vi "Simple Video Analyzer.vi"() -> ()   [LabVIEW 2013]
uses:
  _Type Defs/PhCon GS.ctl
  _Type Defs/PhCon Predefined Cines.ctl
  _Type Defs/PhFile InfName.ctl
  _Type Defs/PHCon IMRANGE.ctl
  _Type Defs/PhInt PhProcessImage Selectors.ctl
  <vilib>/Platform/browser.llb/Open URL in Default Browser (path).vi
  VRI.lvlib
  <vilib>/Analysis/NI_AALBase.lvlib
  _Type Defs/PhCon SDLO.ctl
panel:
  in  "Help":bool
  in  "Exp":dbl format="%#_g us"
  in  "Rate":dbl format="%#_g fps"
  in  "Res":string
  out "Model":string
  out "Image":picture
  out "Frame Brightness":string
  out "Frame":i32(slide) min=-186 max=10 step=1 scale=-2399.0..1999.0
  out "Progress":u8(slide) scale=0.0..100.0
  in  "Save":bool
  in  "Playback":bool
  in  "Trigger":bool
  in  "Record":bool
  out "Name":string
  out "Serial":u32
  in  "Camera Number":u32
  out "IP":string
  # "Simple Video Analyzer"
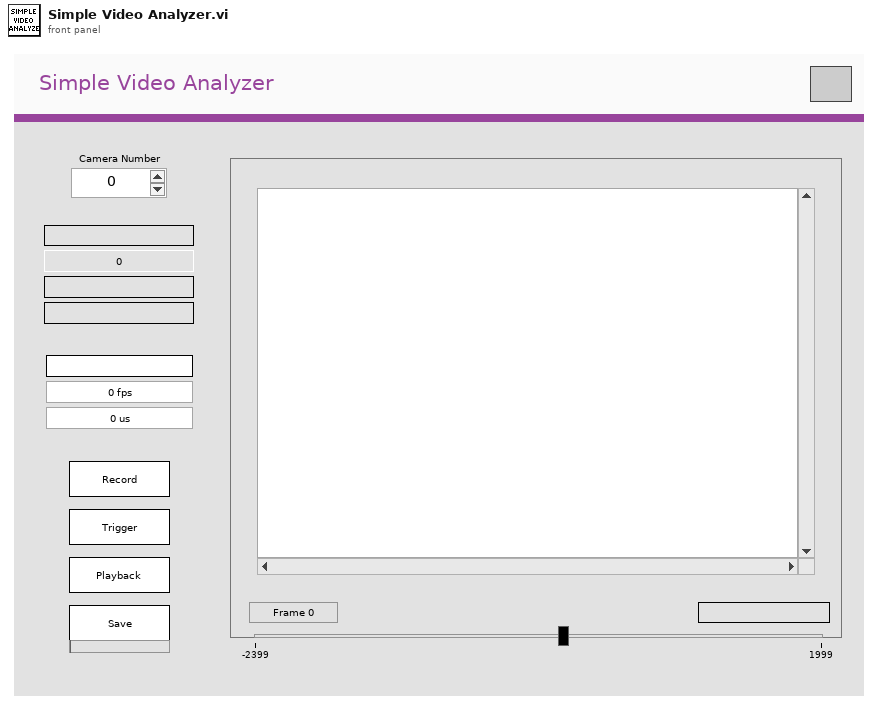
[diagram p1: front panel]
types:
  T1 = typedef "VRI.lvlib/PHCon IMRANGE.ctl" = cluster{"First":i32, "Cnt":u32}
  T2 = typedef "VRI.lvlib/PhCon SDLO.ctl" = u32
  T3 = typedef "VRI.lvlib/PhCon Predefined Cines.ctl" = i32
  T4 = typedef "VRI.lvlib/PhCon GS.ctl" = u16
  T5 = typedef "VRI.lvlib/PHCon ACQUIPARAMS.ctl" = cluster{"ImWidth":u32, "ImHeight":u32, "(deprecated)FrameRateInt":u32, "Exposure":u32, "EDRExposure":u32, "ImDelay":u32, "PTFrames":u32, "ImCount":u32, "SyncImaging":T6, "AutoExposure":u32, "AutoExpLevel":u32, "AutoExpSpeed":u32, "AutoExpRect":T7, "Recorded":bool, "TriggerTime":T8, "RecordedCount":u32, "FirstIm":i32, "FRPSteps":u32, "FRPImgNr":i32[], "FRPRate":u32[], "FRPExp":u32[], "Decimation":u32, "BitDepth":u32, "CamGainRed":u32, "CamGainGreen":u32, "CamGainBlue":u32, "CamGain":u32, "ShutterOff":bool, "CFA":T9, "CineName[256]":u8[], "Description[4096]":u8[], "FRPShape [16]":u32[], "dFrameRate":dbl}
  T6 = typedef "VRI.lvlib/PhCon SyncImaging.ctl" = enum32{"SYNC_INTERNAL", "SYNC_EXTERNAL", "SYNC_LOCKTOIRIG"}
  T7 = typedef "VRI.lvlib/Rect.ctl" = cluster{"X":i32, "Y":i32, "Width":i32, "Height":i32}
  T8 = typedef "VRI.lvlib/PHCon Time64.ctl" = cluster{"fractions":u32, "seconds":u32}
  T9 = typedef "VRI.lvlib/PhInt CFA.ctl" = cluster{"CFA":u32, "VRIV6 Mask":cluster{"TL_GRAY":bool, "TR_GRAY":bool, "BL_GRAY":bool, "BR_GRAY":bool}}
  T10 = typedef "VRI.lvlib/PhFile InfName.ctl" = u32
  T11 = typedef "VRI.lvlib/PhInt PhProcessImage Selectors.ctl" = u16
  T12 = typedef "VRI.lvlib/PhInt IH.ctl" = cluster{"biSize":u32, "biWidth":i32, "biHeight":i32, "biPlanes":u16, "biBitCount":u16, "biCompresssion":u32, "biSizeImage":u32, "biXPelsPerMeter":i32, "biYPelsPerMeter":i32, "biClrUsed":u32, "biClrImportant":u32, "BlackLevel":i32, "WhiteLevel":i32}
  T13 = typedef "VRI.lvlib/BITMAPINFOHEADER.ctl" = cluster{"biSize":u32, "biWidth":i32, "biHeight":i32, "biPlanes":u16, "biBitCount":u16, "biCompression":u32, "biSizeImage":u32, "biXPelsPerMeter":i32, "biYPelsPerMeter":i32, "biClrUsed":u32, "biClrImportant":u32}
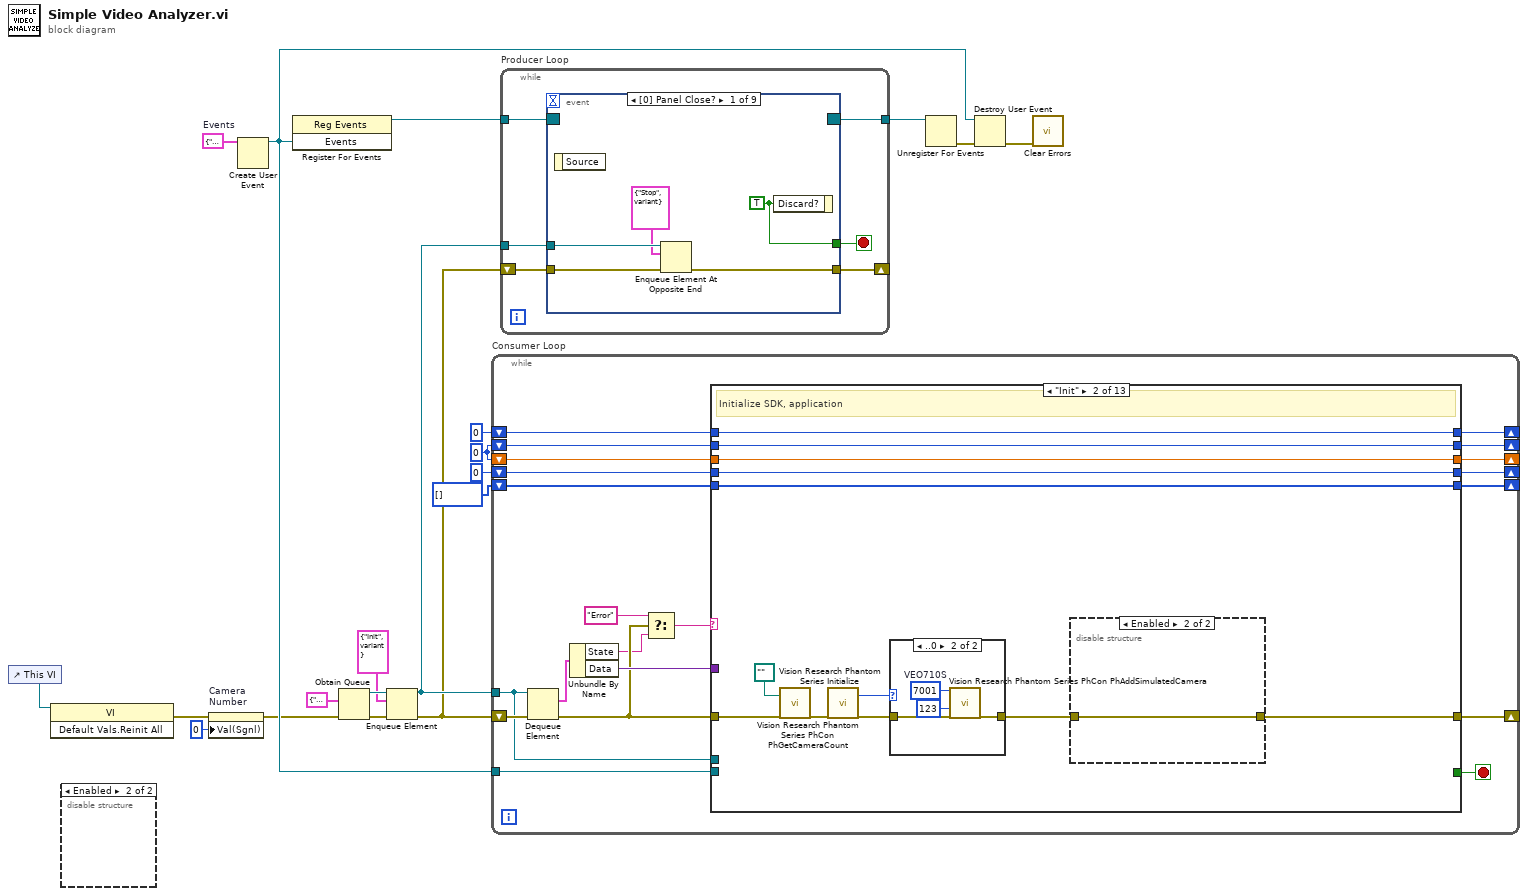
[diagram p0: block diagram]
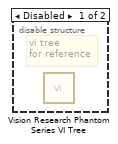
[diagram p2: hidden frame]
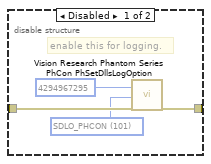
[diagram p5: hidden frame]
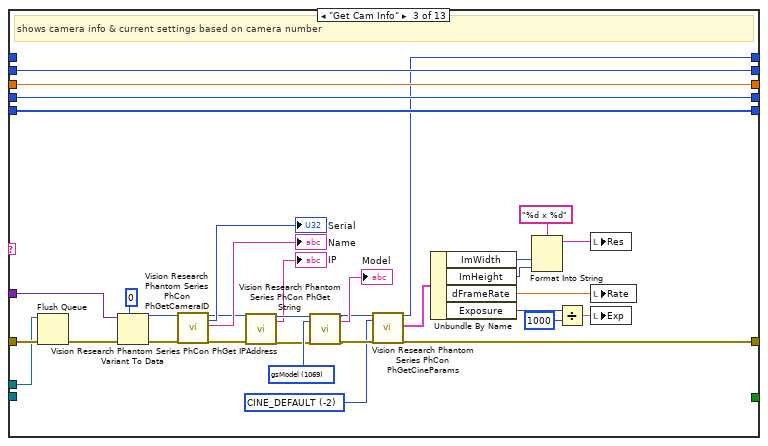
[diagram p6: hidden frame]
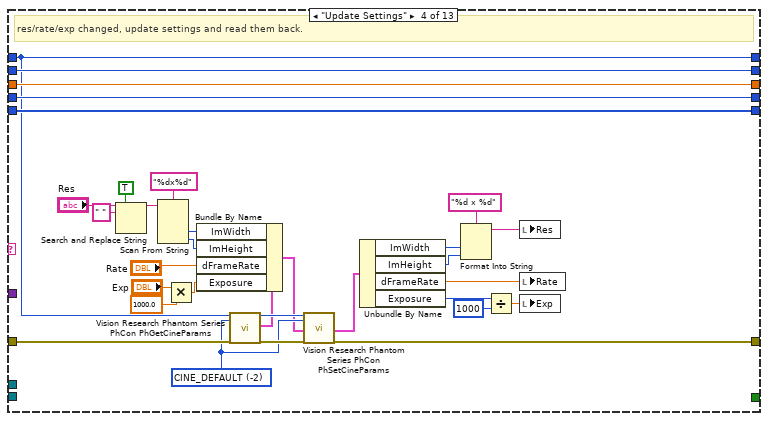
[diagram p7: hidden frame]
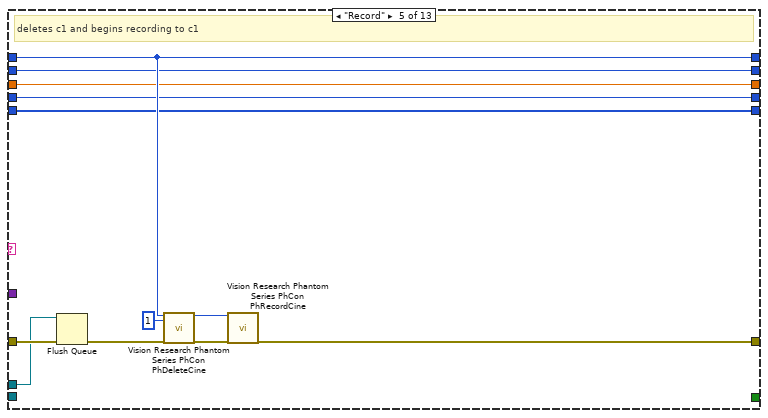
[diagram p8: hidden frame]
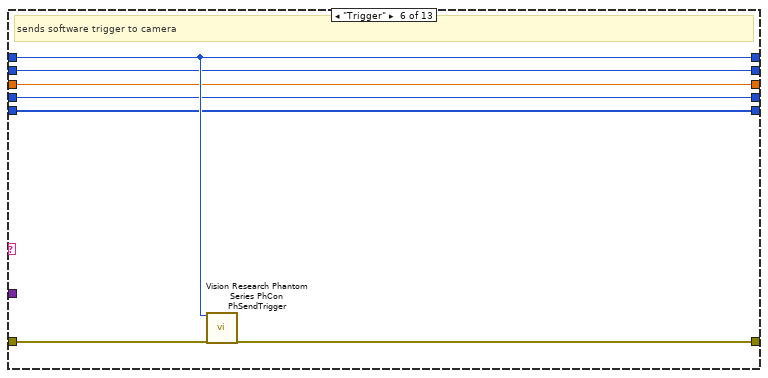
[diagram p9: hidden frame]
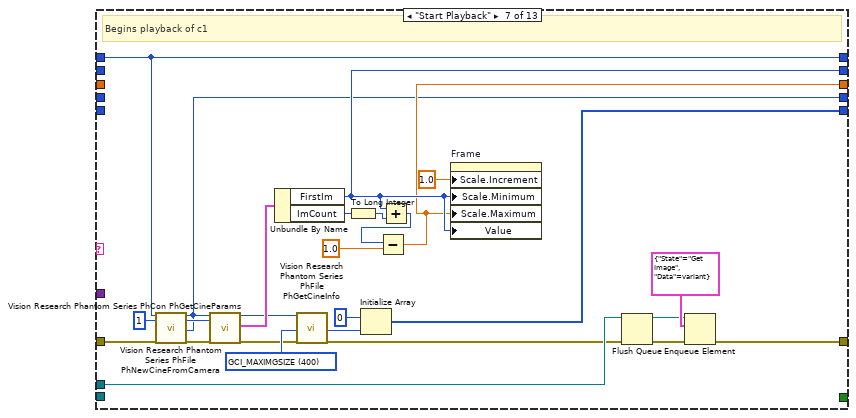
[diagram p10: hidden frame]
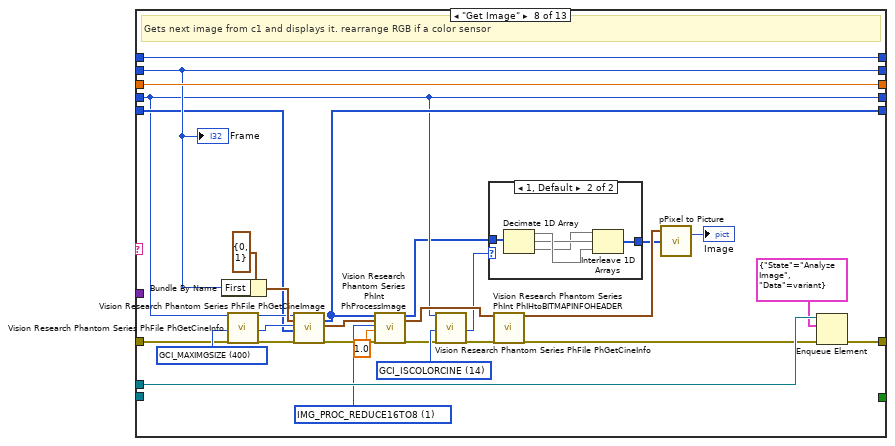
[diagram p11: hidden frame]
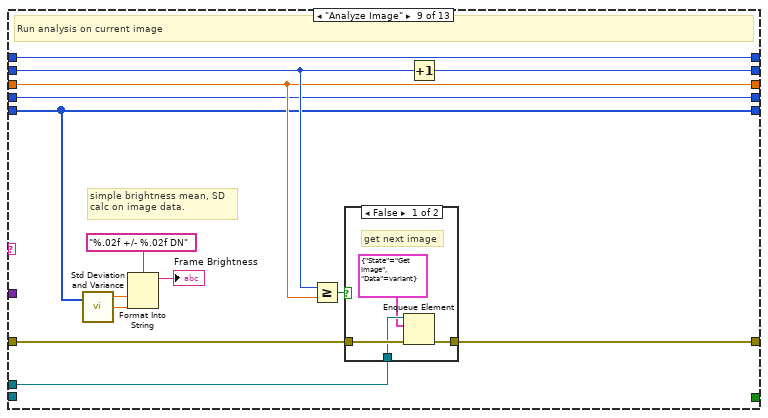
[diagram p13: hidden frame]
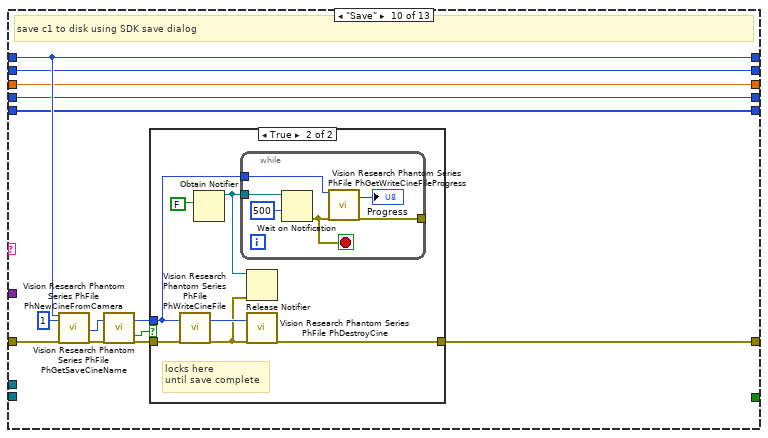
[diagram p15: hidden frame]
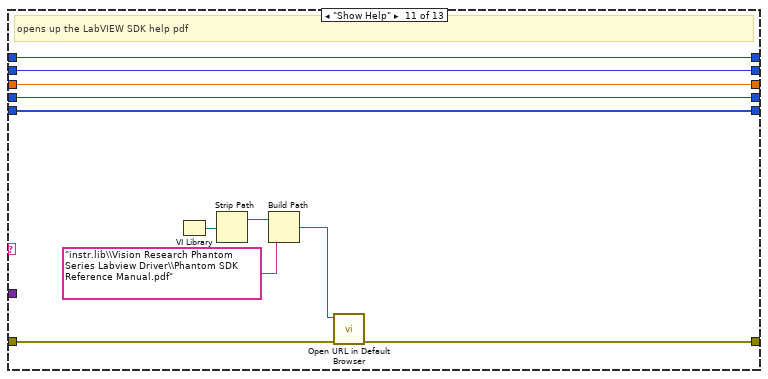
[diagram p17: hidden frame]
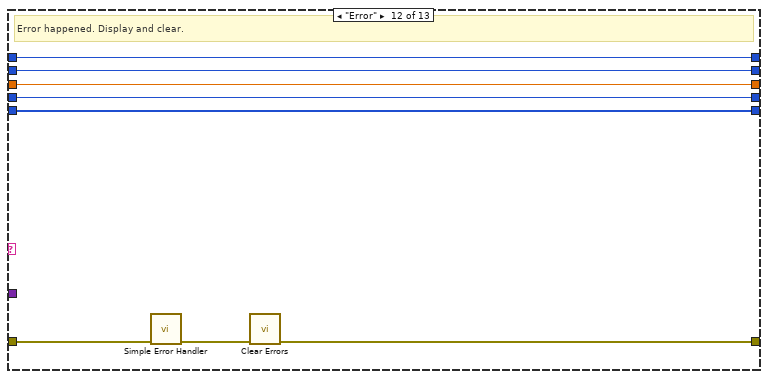
[diagram p18: hidden frame]
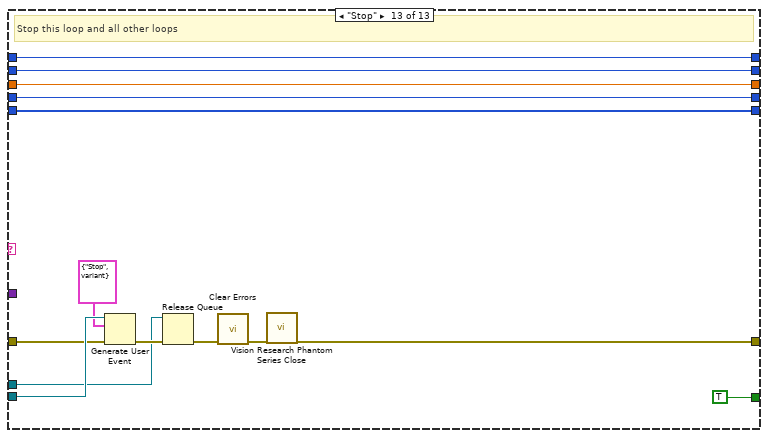
[diagram p19: hidden frame]
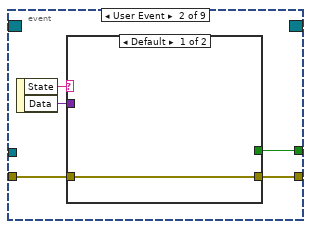
[diagram p20: hidden frame]
diagram:
  w3 = 0 ("CN out")
  w18 = cluster{"State":string, "Data":variant} {"State"="", "Data"=variant}  # Events
  n1 = control-ref of="This VI"() -> (w8:refnum<vi>)
  n2 = invoke class="VI" method="Default Vals.Reinit All"(reference=w8) -> (error out=w6:errorcluster)  [unwired: 2 in, 2 out]
  n3 = disable-structure shown="Enabled" {
    frame Disabled {
      # "vi tree\nfor reference"
      n4 = call "Vision Research Phantom Series VI Tree.vi"() -> ()  [unwired: 12 in]
    }
    frame Enabled {
    }
  }
  n5 = property on="Camera\nNumber" class="DigNum (strict)"(error in=w6, "Val(Sgnl)"=u32 0 ("Value (Signaling)")) -> (error out=w5:errorcluster)  [unwired: 1 in, 1 out]
  n6 = Create User Event(user event datatype=w18) -> (user event=w13:refnum<user-event>)  [unwired: 1 in, 1 out]
  n7 = register-events(w13) -> (reference out=w17:refnum<event-registration>)  [unwired: 2 in, 1 out]
  n8 = Obtain Queue(element data type=cluster{"State":string, "Data":variant} {"State"="", "Data"=variant}, error in (no error)=w5) -> (queue out=w19:refnum<queue>, error out=w11:errorcluster)  [unwired: 3 in, 1 out]
  n9 = Enqueue Element(queue=w19, element=cluster{"State":string, "Data":variant} {"State"="Init", "Data"=variant}, error in (no error)=w11) -> (queue out=w12:refnum<queue>, error out=w10:errorcluster)  [unwired: 1 in, 1 out]
  n10 = while "Consumer Loop" {
    shift-right: [w40] -> _
    shift-left: w10 -> [w41]
    tunnel: w12 -> [w29]
    tunnel: w13 -> [w32]
    shift-right: [w31] -> _
    shift-left: u32 0 ("CN out") -> [w30]
    shift-right: [w28] -> _
    shift-left: w3 -> [w27]
    shift-right: [w26] -> _
    shift-left: w3 -> [w25]
    shift-right: [w24] -> _
    shift-left: u32 0 ("pCH") -> [w23]
    shift-right: [w22] -> _
    shift-left: u16[] [] -> [w21]
    stop <- w33 stop-if-true
    n11 = Dequeue Element(queue=w29, error in (no error)=w41) -> (element=w39:cluster{"State":string, "Data":variant}, error out=w37:errorcluster)  [unwired: 1 in, 2 out]
    n12 = Unbundle By Name(w39) -> ("State"=w36:string, "Data"=w38:variant)
    n13 = Select(t="Error", s=w37, f=w36) -> (s? t:f=w35:string)
    n14 = case shown="\"Init\"" w35 {
      tunnel: w37 -> [w47 w59 w103 w122 w138 w154 w177 w205 w230 w248 w273 w281 w290]
      tunnel: [w47 w53 w75 w131 w147 w153 w173 w209 w228 w242 w272 w279 w289] -> w40
      tunnel: w29 -> [_ _ w70 _ w136 _ w167 w208 w227 _ _ _ w286]
      tunnel: w38 -> [_ _ w102 _ _ _ _ _ _ _ _ _ _]
      tunnel: [_ _ _ _ _ _ _ _ _ _ _ _ TRUE] -> w33
      tunnel: w32 -> [_ _ _ _ _ _ _ _ _ _ _ _ w294]
      tunnel: [w46 w58 w73 w120 w145 w152 w176 w210 w229 w247 w271 w278 w288] -> w31
      tunnel: w30 -> [w46 w58 _ w120 w145 w152 w176 w210 w229 w247 w271 w278 w288]
      tunnel: [w45 w57 w97 w135 w142 w151 w164 w200 w223 w239 w270 w277 w285] -> w28
      tunnel: w27 -> [w45 w57 w97 w135 w142 w151 _ w200 w225 w239 w270 w277 w285]
      tunnel: [w44 w56 w96 w134 w141 w150 w161 w207 w224 w238 w269 w276 w284] -> w26
      tunnel: w25 -> [w44 w56 w96 w134 w141 w150 _ w207 w224 w238 w269 w276 w284]
      tunnel: [w43 w55 w95 w133 w140 w149 w158 w186 w222 w237 w268 w275 w283] -> w24
      tunnel: w23 -> [w43 w55 w95 w133 w140 w149 _ w186 w222 w237 w268 w275 w283]
      tunnel: [w42 w54 w94 w132 w139 w148 w168 w194 w221 w236 w267 w274 w282] -> w22
      tunnel: w21 -> [w42 w54 w94 w132 w139 w148 _ w198 w221 w236 w267 w274 w282]
      frame Default {
      }
      frame "Init" {
        # "Initialize SDK, application"
        n15 = call "Vision Research Phantom Series Initialize.vi"("Storage Path (\"\")"=path "" ("Storage Path (\"\")"), "error in (no error)"=w59) -> ("Error Out"=w52:errorcluster)  [unwired: 16 in, 1 out]
        n16 = call "Vision Research Phantom Series PhCon PhGetCameraCount.vi"("Error In (no error)"=w52) -> ("pCnt"=w49:u32, "Error Out"=w51:errorcluster)  [unwired: 17 in]
        n17 = case shown="..0" w49 {
          tunnel: w51 -> [w60 w64]
          tunnel: [w60 w63] -> w50
          frame 1.. {
          }
          frame ..0 {
            w62 = u32 7001  # VEO710S
            n18 = call "Vision Research Phantom Series PhCon PhAddSimulatedCamera.vi"("CamVer (in)"=w62, "Serial (in)"=u32 123, "Error In (no error)"=w64) -> ("Error Out"=w63:errorcluster)  [unwired: 16 in]
          }
        }
        n19 = disable-structure shown="Enabled" {
          disable-tunnel: w50 -> [w68 w69]
          disable-tunnel: [w67 w69] -> w53
          frame Disabled {
            w66 = T2 101 items=["SDLO_PHANTOM"=100, "SDLO_PHCON"=101, "SDLO_PHINT"=102, "SDLO_PHFILE"=103, "SDLO_PHSIG"=104, "SDLO_PHSIGV"=105, "SDLO_TORAM"=106] ("SelectCode")
            # "enable this for logging."
            n20 = call "Vision Research Phantom Series PhCon PhSetDllsLogOption.vi"("Value"=u32 4294967295, "SelectCode"=w66, "Error In (no error)"=w68) -> ("Error Out"=w67:errorcluster)  [unwired: 16 in]
          }
          frame Enabled {
          }
        }
      }
      frame "Get Cam Info" {
        w72 = T3 -2 items=["CINE_DEFAULT "=-2, "CINE_CURRENT "=-1, "CINE_PREVIEW  "=0, "CINE_FIRST    "=1, "FIRST_FLASH_CINE"=101] ("Cine")
        w92 = T4 1069 items=["gsHasMechanicalShutter"=1025, "gsHasBlackLevel4"=1027, "gsHasCardFlash"=1051, "gsHas10G"=2000, "gsSupportsInternalBlackRef"=1026, "gsSupportsImageTrig"=1040, "gsSupportsCardFlash"=1050, "gsSupportsMagazine"=8193, "gsSupportsHQMode"=8194, "gsSupportsGenlock"=8195, "gsSupportsEDR"=8196, "gsSupportsAutoExposure"=8197, "gsSupportsTurbo"=8198, "gsSupportsBurstMode"=8199, "gsSupportsShutterOff"=8200, "gsSupportsDualSDIOutput"=8201, "gsSupportsRecordingCines"=8202, "gsSupportsV444"=8203, "gsSupportsInterlacedSensor"=8204, "gsSupportsRampFRP"=8205, "gsSensorTemperature"=1028, "gsCameraTemperature"=1029, "gsThermoElectricPower"=1030, "gsSensorTemperatureThreshold"=1031, "gsCameraTemperatureThreshold"=1032, "gsVideoPlayCine"=1033, "gsVideoPlaySpeed"=1034, "gsVideoOutputConfig"=1035, "gsMechanicalShutter"=1036, "gsImageTrigThreshold"=1041, "gsImageTrigAreaPercentage"=1042, "gsImageTrigSpeed"=1043, "gsImageTrigMode"=1044, "gsImageTrigRect"=1045, "gsAutoProgress"=1046, "gsAutoBlackRef"=1047, "gsCardFlashSizeK"=1052, "gsCardFlashFreeK"=1053, "gsCardFlashError"=1054, "gsEthernetAddress"=1055, "gsEthernetMask"=1056, "gsEthernetBroadcast"=1057, "gsEthernetGateway"=1058, "gsLensFocus"=1059, "gsLensAperature"=1060, "gsLensAperatureRange"=1061, "gsLensDescription"=1062, "gsLensFocusInProgress"=1063, "gsLensFocusAtLimit"=1064, "gsGenlock"=1065, "gsGenlockStatus"=1066, "gsTurboMode"=1068, "gsModel"=1069, "gsIPAddress"=1070] ("Sel")
        # "shows camera info & current settings based on camera number"
        n21 = Flush Queue(queue=w70, error in (no error)=w103) -> (error out=w71:errorcluster)  [unwired: 2 out]
        n22 = Variant To Data(error in=w71, type=u32 0, Variant=w102) -> (data=w99:u32, error out=w100:errorcluster)
        n23 = call "Vision Research Phantom Series PhCon PhGetCameraID.vi"("CN in"=w99, "Error In (no error)"=w100) -> ("CN out"=w90:u32, "pSerial"=→"Serial":u32, "pCameraName"=→"Name":string, "Error Out"=w88:errorcluster)  [unwired: 14 in]
        n24 = call "Vision Research Phantom Series PhCon PhGet IPAddress.vi"("CN [in]"=w90, "Error In (no error)"=w88) -> ("CN [out]"=w89:u32, "IP Address"=→"IP":string, "Error Out"=w87:errorcluster)  [unwired: 15 in]
        n25 = call "Vision Research Phantom Series PhCon PhGet String.vi"("CN [in]"=w89, "Sel"=w92, "Error In (no error)"=w87) -> ("CN [out]"=w74:u32, "pVal [out]"=→"Model":string, "Error Out"=w76:errorcluster)  [unwired: 14 in]
        n26 = call "Vision Research Phantom Series PhCon PhGetCineParams.vi"("CN in"=w74, "Cine"=w72, "Error In (no error)"=w76) -> ("CN out"=w73:u32, "ACQUIPARAMS"=w85:T5, "Error Out"=w75:errorcluster)  [unwired: 14 out]
        n27 = Unbundle By Name(w85) -> ("ImWidth"=w84:u32, "ImHeight"=w83:u32, "dFrameRate"=w80:dbl, "Exposure"=w78:u32)
        n28 = Format Into String(format string="%d x %d", w84, w83) -> (resulting string=w81:string)  [unwired: 2 in, 1 out]
        n29 = Divide(x=w78, y=u32 1000) -> (x/y=w79:dbl)
        n30 = local write "Res"(w81) -> ()
        n31 = local write "Rate"(w80) -> ()
        n32 = local write "Exp"(w79) -> ()
      }
      frame "Update Settings" {
        w118 = T3 -2 items=["CINE_DEFAULT "=-2, "CINE_CURRENT "=-1, "CINE_PREVIEW  "=0, "CINE_FIRST    "=1, "FIRST_FLASH_CINE"=101] ("Cine")
        # "res/rate/exp changed, update settings and read them back."
        n33 = Search and Replace String(replace all?=TRUE ("replace all? (F)"), input string="Res", search string=" ") -> (result string=w109:string)  [unwired: 5 in, 3 out]
        n34 = Scan From String(format string="%dx%d", input string=w109) -> (output 1=w105:i32, output 2=w104:i32)  [unwired: 4 in, 3 out]
        n35 = Multiply(x="Exp", y=1000.0) -> (x*y=w113:dbl)
        n36 = call "Vision Research Phantom Series PhCon PhGetCineParams.vi"("CN in"=w120, "Cine"=w118, "Error In (no error)"=w122) -> ("CN out"=w119:u32, "ACQUIPARAMS"=w117:T5, "Error Out"=w121:errorcluster)  [unwired: 14 out]
        n37 = Bundle By Name(cluster=w117, "ImWidth"=w105, "ImHeight"=w104, "dFrameRate"="Rate", "Exposure"=w113) -> (w116:T5)
        n38 = call "Vision Research Phantom Series PhCon PhSetCineParams.vi"("CN in"=w119, "Cine"=w118, "ACQUIPARAMS"=w116, "Error In (no error)"=w121) -> ("ACQUIPARAMS out"=w111:T5, "Error Out"=w131:errorcluster)  [unwired: 14 out]
        n39 = Unbundle By Name(w111) -> ("ImWidth"=w130:u32, "ImHeight"=w129:u32, "dFrameRate"=w126:dbl, "Exposure"=w124:u32)
        n40 = Format Into String(format string="%d x %d", w130, w129) -> (resulting string=w127:string)  [unwired: 2 in, 1 out]
        n41 = Divide(x=w124, y=u32 1000) -> (x/y=w125:dbl)
        n42 = local write "Res"(w127) -> ()
        n43 = local write "Rate"(w126) -> ()
        n44 = local write "Exp"(w125) -> ()
      }
      frame "Record" {
        # "deletes c1 and begins recording to c1"
        n45 = Flush Queue(queue=w136, error in (no error)=w138) -> (error out=w137:errorcluster)  [unwired: 2 out]
        n46 = call "Vision Research Phantom Series PhCon PhDeleteCine.vi"("CN in"=w145, "Cine"=1, "Error In (no error)"=w137) -> ("CN out"=w144:u32, "Error Out"=w146:errorcluster)  [unwired: 15 out]
        n47 = call "Vision Research Phantom Series PhCon PhRecordCine.vi"("CN in"=w144, "Error In (no error)"=w146) -> ("Error Out"=w147:errorcluster)  [unwired: 17 out]
      }
      frame "Trigger" {
        # "sends software trigger to camera"
        n48 = call "Vision Research Phantom Series PhCon PhSendTrigger.vi"("CN in"=w152, "Error In (no error)"=w154) -> ("Error Out"=w153:errorcluster)  [unwired: 17 out]
      }
      frame "Start Playback" {
        w159 = T10 400 items=["GCI_CFA"=0, "GCI_FRAMERATE"=1, "GCI_EXPOSURE"=2, "GCI_AUTOEXPOSURE"=3, "GCI_REALBPP"=4, "GCI_CAMERASERIAL"=5, "GCI_HEADSERIAL0"=6, "GCI_HEADSERIAL1"=7, "GCI_HEADSERIAL2"=8, "GCI_HEADSERIAL3"=9, "GCI_TRIGTIMESEC"=10, "GCI_TRIGTIMEFR"=11, "GCI_ISFILECINE"=12, "GCI_IS16BPPCINE"=13, "GCI_ISCOLORCINE"=14, "GCI_ISMULTIHEADCINE"=15, "GCI_EXPOSURENS"=16, "GCI_EDREXPOSURENS"=17, "GCI_FRAMEDELAYNS"=19, "GCI_FROMFILETYPE"=20, "GCI_COMPRESSION"=21, "GCI_CAMERAVERSION"=22, "GCI_ROTATE"=23, "GCI_IMWIDTH"=24, "GCI_IMHEIGHT"=25, "GCI_IMWIDTHACQ"=26, "GCI_IMHEIGHTACQ"=27, "GCI_POSTTRIGGER"=28, "GCI_IMAGECOUNT"=29, "GCI_TOTALIMAGECOUNT"=30, "GCI_TRIGFRAME"=31, "GCI_AUTOEXPLEVEL"=32, "GCI_AUTOEXPTOP"=33, "GCI_AUTOEXPLEFT"=34, "GCI_AUTOEXPBOTTOM"=35, "GCI_AUTOEXPRIGHT"=36, "GCI_RECORDINGTIMEZONE"=37, "GCI_FIRSTIMAGENO"=38, "GCI_FIRSTMOVIEIMAGE"=39, "GCI_CINENAME"=40, "GCI_FRPSTEPS"=100, "GCI_FRP1X"=101, "GCI_FRP1Y"=102, "GCI_FRP2X"=103, "GCI_FRP2Y"=104, "GCI_FRP3X"=105, "GCI_FRP3Y"=106, "GCI_FRP4X"=107, "GCI_FRP4Y"=108, "GCI_WRITEERR"=109, "GCI_LENSDESCRIPTION"=110, "GCI_LENSAPERATURE"=111, "GCI_LENSFOCALLENGTH"=112, "GCI_WB"=200, "GCI_WBVIEW"=201, "GCI_BRIGHT"=202, "GCI_CONTRAST"=203, "GCI_GAMMA"=204, "GCI_GAMMAR"=223, "GCI_GAMMAB"=224, "GCI_SATURATION"=205, "GCI_HUE"=206, "GCI_FLIPH"=207, "GCI_FLIPV"=208, "GCI_FILTERCODE"=209, "GCI_IMFILTER"=210, "GCI_INTALGO"=211, "GCI_PEDESTALR"=212, "GCI_PEDESTALG"=213, "GCI_PEDESTALB"=214, "GCI_FLARE"=225, "GCI_CHROMA"=226, "GCI_TONE"=227, "GCI_ENABLEMATRICES"=228, "GCI_USERMATRIX"=229, "GCI_RESAMPLEACTIVE"=215, "GCI_RESAMPLEWIDTH"=216, "GCI_RESAMPLEHEIGHT"=217, "GCI_CROPACTIVE"=218, "GCI_CROPRECTANGLE"=219, "GCI_OFFSET16_8"=220, "GCI_GAIN16_8"=221, "GCI_DEMOSAICINGFUNCPTR"=222, "GCI_VFLIPVIEWACTIVE"=300, "GCI_MAXIMGSIZE"=400, "GCI_FRPIMGNOARRAY"=450, "GCI_FRPRATEARRAY"=451, "GCI_FRPSHAPEARRAY"=452, "GCI_TRIGTC"=470, "GCI_TRIGTCU"=471, "GCI_PBRATE"=472, "GCI_TCRATE"=473, "GCI_SAVERANGE"=500, "GCI_SAVEFILENAME"=501, "GCI_SAVEFILETYPE"=502, "GCI_SAVE16BIT"=503, "GCI_SAVEPACKED"=504, "GCI_SAVEXML"=505, "GCI_SAVESTAMPTIME"=506, "GCI_SAVEAVIFRAMERATE"=520, "GCI_SAVEAVICOMPRESSORLIST"=521, "GCI_SAVEAVICOMPRESSORINDEX"=522, "GCI_SAVEDPXLSB"=530, "GCI_SAVEDPXTO10BPS"=531, "GCI_SAVEDPXDATAPACKING"=532, "GCI_SAVEDPX10BITLOG"=533, "GCI_SAVEDPXEXPORTLOGLUT"=534, "GCI_SAVEDPX10BITLOGREFWHITE"=535, "GCI_SAVEDPX10BITLOGREFBLACK"=536, "GCI_SAVEDPX10BITLOGGAMMA"=537, "GCI_SAVEDPX10BITLOGFILMGAMMA"=538, "GCI_SAVEQTPLAYBACKRATE"=550, "GCI_SAVECCIQUALITY"=560, "GCI_UNCALIBRATEDIMAGE"=600, "GCI_NOPROCESSING"=601, "GCI_BADPIXELREPAIR"=602] ("InfName")
        # "Begins playback of c1"
        n49 = call "Vision Research Phantom Series PhFile PhNewCineFromCamera.vi"("Camera Number in"=w176, "CineNr in"=1, "Error In (no error)"=w177) -> ("Camera Number out"=w180:u32, "CineNr out"=w179:i32, "pCH"=w158:u32, "Error Out"=w160:errorcluster)  [unwired: 1 in, 12 out]
        n50 = call "Vision Research Phantom Series PhCon PhGetCineParams.vi"("CN in"=w180, "Cine"=w179, "Error In (no error)"=w160) -> ("ACQUIPARAMS"=w175:T5, "Error Out"=w157:errorcluster)  [unwired: 15 out]
        n51 = Unbundle By Name(w175) -> ("FirstIm"=w164:i32, "ImCount"=w174:u32)
        n52 = call "Vision Research Phantom Series PhFile PhGetCineInfo.vi"("CH in"=w158, "InfName"=w159, "Error In (no error)"=w157) -> ("pInfVal out"=w155:i32, "Error Out"=w156:errorcluster)  [unwired: 15 out]
        n53 = To Long Integer(number=w174) -> (32bit integer=w170:i32)
        n54 = Initialize Array(u16 0 ("element"), w155) -> (w168:u16[])
        n55 = Add(x=w164, y=w170) -> (x+y=w162:i32)
        n56 = Subtract(x=w162, y=1.0 ("Scale.Range:Increment")) -> (x-y=w161:dbl)
        n57 = property on="Frame" class="Slide (strict)"("Scale.Increment"=1.0 ("Scale.Range:Increment"), "Scale.Minimum"=w164, "Scale.Maximum"=w161, "Value"=w164) -> ()  [unwired: 2 in, 2 out]
        n58 = Flush Queue(queue=w167, error in (no error)=w156) -> (queue out=w165:refnum<queue>, error out=w166:errorcluster)  [unwired: 1 out]
        n59 = Enqueue Element(queue=w165, element=cluster{"State":string, "Data":variant} {"State"="Get Image", "Data"=variant}, error in (no error)=w166) -> (error out=w173:errorcluster)  [unwired: 1 in, 2 out]
      }
      frame "Get Image" {
        w188 = T10 14 items=["GCI_CFA"=0, "GCI_FRAMERATE"=1, "GCI_EXPOSURE"=2, "GCI_AUTOEXPOSURE"=3, "GCI_REALBPP"=4, "GCI_CAMERASERIAL"=5, "GCI_HEADSERIAL0"=6, "GCI_HEADSERIAL1"=7, "GCI_HEADSERIAL2"=8, "GCI_HEADSERIAL3"=9, "GCI_TRIGTIMESEC"=10, "GCI_TRIGTIMEFR"=11, "GCI_ISFILECINE"=12, "GCI_IS16BPPCINE"=13, "GCI_ISCOLORCINE"=14, "GCI_ISMULTIHEADCINE"=15, "GCI_EXPOSURENS"=16, "GCI_EDREXPOSURENS"=17, "GCI_FRAMEDELAYNS"=19, "GCI_FROMFILETYPE"=20, "GCI_COMPRESSION"=21, "GCI_CAMERAVERSION"=22, "GCI_ROTATE"=23, "GCI_IMWIDTH"=24, "GCI_IMHEIGHT"=25, "GCI_IMWIDTHACQ"=26, "GCI_IMHEIGHTACQ"=27, "GCI_POSTTRIGGER"=28, "GCI_IMAGECOUNT"=29, "GCI_TOTALIMAGECOUNT"=30, "GCI_TRIGFRAME"=31, "GCI_AUTOEXPLEVEL"=32, "GCI_AUTOEXPTOP"=33, "GCI_AUTOEXPLEFT"=34, "GCI_AUTOEXPBOTTOM"=35, "GCI_AUTOEXPRIGHT"=36, "GCI_RECORDINGTIMEZONE"=37, "GCI_FIRSTIMAGENO"=38, "GCI_FIRSTMOVIEIMAGE"=39, "GCI_CINENAME"=40, "GCI_FRPSTEPS"=100, "GCI_FRP1X"=101, "GCI_FRP1Y"=102, "GCI_FRP2X"=103, "GCI_FRP2Y"=104, "GCI_FRP3X"=105, "GCI_FRP3Y"=106, "GCI_FRP4X"=107, "GCI_FRP4Y"=108, "GCI_WRITEERR"=109, "GCI_LENSDESCRIPTION"=110, "GCI_LENSAPERATURE"=111, "GCI_LENSFOCALLENGTH"=112, "GCI_WB"=200, "GCI_WBVIEW"=201, "GCI_BRIGHT"=202, "GCI_CONTRAST"=203, "GCI_GAMMA"=204, "GCI_GAMMAR"=223, "GCI_GAMMAB"=224, "GCI_SATURATION"=205, "GCI_HUE"=206, "GCI_FLIPH"=207, "GCI_FLIPV"=208, "GCI_FILTERCODE"=209, "GCI_IMFILTER"=210, "GCI_INTALGO"=211, "GCI_PEDESTALR"=212, "GCI_PEDESTALG"=213, "GCI_PEDESTALB"=214, "GCI_FLARE"=225, "GCI_CHROMA"=226, "GCI_TONE"=227, "GCI_ENABLEMATRICES"=228, "GCI_USERMATRIX"=229, "GCI_RESAMPLEACTIVE"=215, "GCI_RESAMPLEWIDTH"=216, "GCI_RESAMPLEHEIGHT"=217, "GCI_CROPACTIVE"=218, "GCI_CROPRECTANGLE"=219, "GCI_OFFSET16_8"=220, "GCI_GAIN16_8"=221, "GCI_DEMOSAICINGFUNCPTR"=222, "GCI_VFLIPVIEWACTIVE"=300, "GCI_MAXIMGSIZE"=400, "GCI_FRPIMGNOARRAY"=450, "GCI_FRPRATEARRAY"=451, "GCI_FRPSHAPEARRAY"=452, "GCI_TRIGTC"=470, "GCI_TRIGTCU"=471, "GCI_PBRATE"=472, "GCI_TCRATE"=473, "GCI_SAVERANGE"=500, "GCI_SAVEFILENAME"=501, "GCI_SAVEFILETYPE"=502, "GCI_SAVE16BIT"=503, "GCI_SAVEPACKED"=504, "GCI_SAVEXML"=505, "GCI_SAVESTAMPTIME"=506, "GCI_SAVEAVIFRAMERATE"=520, "GCI_SAVEAVICOMPRESSORLIST"=521, "GCI_SAVEAVICOMPRESSORINDEX"=522, "GCI_SAVEDPXLSB"=530, "GCI_SAVEDPXTO10BPS"=531, "GCI_SAVEDPXDATAPACKING"=532, "GCI_SAVEDPX10BITLOG"=533, "GCI_SAVEDPXEXPORTLOGLUT"=534, "GCI_SAVEDPX10BITLOGREFWHITE"=535, "GCI_SAVEDPX10BITLOGREFBLACK"=536, "GCI_SAVEDPX10BITLOGGAMMA"=537, "GCI_SAVEDPX10BITLOGFILMGAMMA"=538, "GCI_SAVEQTPLAYBACKRATE"=550, "GCI_SAVECCIQUALITY"=560, "GCI_UNCALIBRATEDIMAGE"=600, "GCI_NOPROCESSING"=601, "GCI_BADPIXELREPAIR"=602] ("InfName")
        w192 = T11 1 items=["IMG_PROC_REDUCE16TO8"=1] ("procID")
        w206 = T10 400 items=["GCI_CFA"=0, "GCI_FRAMERATE"=1, "GCI_EXPOSURE"=2, "GCI_AUTOEXPOSURE"=3, "GCI_REALBPP"=4, "GCI_CAMERASERIAL"=5, "GCI_HEADSERIAL0"=6, "GCI_HEADSERIAL1"=7, "GCI_HEADSERIAL2"=8, "GCI_HEADSERIAL3"=9, "GCI_TRIGTIMESEC"=10, "GCI_TRIGTIMEFR"=11, "GCI_ISFILECINE"=12, "GCI_IS16BPPCINE"=13, "GCI_ISCOLORCINE"=14, "GCI_ISMULTIHEADCINE"=15, "GCI_EXPOSURENS"=16, "GCI_EDREXPOSURENS"=17, "GCI_FRAMEDELAYNS"=19, "GCI_FROMFILETYPE"=20, "GCI_COMPRESSION"=21, "GCI_CAMERAVERSION"=22, "GCI_ROTATE"=23, "GCI_IMWIDTH"=24, "GCI_IMHEIGHT"=25, "GCI_IMWIDTHACQ"=26, "GCI_IMHEIGHTACQ"=27, "GCI_POSTTRIGGER"=28, "GCI_IMAGECOUNT"=29, "GCI_TOTALIMAGECOUNT"=30, "GCI_TRIGFRAME"=31, "GCI_AUTOEXPLEVEL"=32, "GCI_AUTOEXPTOP"=33, "GCI_AUTOEXPLEFT"=34, "GCI_AUTOEXPBOTTOM"=35, "GCI_AUTOEXPRIGHT"=36, "GCI_RECORDINGTIMEZONE"=37, "GCI_FIRSTIMAGENO"=38, "GCI_FIRSTMOVIEIMAGE"=39, "GCI_CINENAME"=40, "GCI_FRPSTEPS"=100, "GCI_FRP1X"=101, "GCI_FRP1Y"=102, "GCI_FRP2X"=103, "GCI_FRP2Y"=104, "GCI_FRP3X"=105, "GCI_FRP3Y"=106, "GCI_FRP4X"=107, "GCI_FRP4Y"=108, "GCI_WRITEERR"=109, "GCI_LENSDESCRIPTION"=110, "GCI_LENSAPERATURE"=111, "GCI_LENSFOCALLENGTH"=112, "GCI_WB"=200, "GCI_WBVIEW"=201, "GCI_BRIGHT"=202, "GCI_CONTRAST"=203, "GCI_GAMMA"=204, "GCI_GAMMAR"=223, "GCI_GAMMAB"=224, "GCI_SATURATION"=205, "GCI_HUE"=206, "GCI_FLIPH"=207, "GCI_FLIPV"=208, "GCI_FILTERCODE"=209, "GCI_IMFILTER"=210, "GCI_INTALGO"=211, "GCI_PEDESTALR"=212, "GCI_PEDESTALG"=213, "GCI_PEDESTALB"=214, "GCI_FLARE"=225, "GCI_CHROMA"=226, "GCI_TONE"=227, "GCI_ENABLEMATRICES"=228, "GCI_USERMATRIX"=229, "GCI_RESAMPLEACTIVE"=215, "GCI_RESAMPLEWIDTH"=216, "GCI_RESAMPLEHEIGHT"=217, "GCI_CROPACTIVE"=218, "GCI_CROPRECTANGLE"=219, "GCI_OFFSET16_8"=220, "GCI_GAIN16_8"=221, "GCI_DEMOSAICINGFUNCPTR"=222, "GCI_VFLIPVIEWACTIVE"=300, "GCI_MAXIMGSIZE"=400, "GCI_FRPIMGNOARRAY"=450, "GCI_FRPRATEARRAY"=451, "GCI_FRPSHAPEARRAY"=452, "GCI_TRIGTC"=470, "GCI_TRIGTCU"=471, "GCI_PBRATE"=472, "GCI_TCRATE"=473, "GCI_SAVERANGE"=500, "GCI_SAVEFILENAME"=501, "GCI_SAVEFILETYPE"=502, "GCI_SAVE16BIT"=503, "GCI_SAVEPACKED"=504, "GCI_SAVEXML"=505, "GCI_SAVESTAMPTIME"=506, "GCI_SAVEAVIFRAMERATE"=520, "GCI_SAVEAVICOMPRESSORLIST"=521, "GCI_SAVEAVICOMPRESSORINDEX"=522, "GCI_SAVEDPXLSB"=530, "GCI_SAVEDPXTO10BPS"=531, "GCI_SAVEDPXDATAPACKING"=532, "GCI_SAVEDPX10BITLOG"=533, "GCI_SAVEDPXEXPORTLOGLUT"=534, "GCI_SAVEDPX10BITLOGREFWHITE"=535, "GCI_SAVEDPX10BITLOGREFBLACK"=536, "GCI_SAVEDPX10BITLOGGAMMA"=537, "GCI_SAVEDPX10BITLOGFILMGAMMA"=538, "GCI_SAVEQTPLAYBACKRATE"=550, "GCI_SAVECCIQUALITY"=560, "GCI_UNCALIBRATEDIMAGE"=600, "GCI_NOPROCESSING"=601, "GCI_BADPIXELREPAIR"=602] ("InfName")
        # "Gets next image from c1 and displays it. rearrange RGB if a color sensor"
        n60 = Bundle By Name(cluster=T1 {"First"=0, "Cnt"=1} ("pRng"), "First"=w200) -> (w203:T1)
        n61 = call "Vision Research Phantom Series PhFile PhGetCineInfo.vi"("CH in"=w186, "InfName"=w206, "Error In (no error)"=w205) -> ("CH out"=w201:u32, "pInfVal out"=w199:i32, "Error Out"=w204:errorcluster)  [unwired: 14 out]
        n62 = call "Vision Research Phantom Series PhFile PhGetCineImage.vi"("hC [in]"=w201, "pRng [in]"=w203, "bufferByteSize [in]"=w199, "pPixelBuffer [in]"=w198, "Error In (no error)"=w204) -> ("pPixelBuffer [out]"=w194:u16[], "IH [out]"=w191:T12, "Error Out"=w193:errorcluster)  [unwired: 12 out]
        n63 = call "Vision Research Phantom Series PhInt PhProcessImage.vi"("pPixelSrc [in]"=w194, "IH [in]"=w191, "procID"=w192, "pProcParams"=1.0, "Error In (no error)"=w193) -> ("pPixelDest [out]"=w183:u8[], "IH [out]"=w196:T12, "Error Out"=w187:errorcluster)  [unwired: 12 out]
        n64 = call "Vision Research Phantom Series PhFile PhGetCineInfo.vi"("CH in"=w186, "InfName"=w188, "Error In (no error)"=w187) -> ("pInfVal out"=w182:i32, "Error Out"=w185:errorcluster)  [unwired: 15 out]
        n65 = case shown="1, Default" w182 {
          tunnel: w183 -> [w211 w212]
          tunnel: [w211 w213] -> w184
          frame 0 {
          }
          frame 1, Default {
            n66 = Decimate 1D Array(w212) -> (w216:u8[], w215:u8[], w214:u8[])
            n67 = Interleave 1D Arrays(w214, w215, w216) -> (w213:u8[])
          }
        }
        n68 = call "Vision Research Phantom Series PhInt PhIHtoBITMAPINFOHEADER.vi"("IH"=w196, "Error In (no error)"=w185) -> ("BITMAPINFOHEADER"=w197:T13, "Error Out"=w189:errorcluster)  [unwired: 16 out]
        n69 = call "pPixel to Picture.vi"("pPixel"=w184, "BITMAPINFOHEADER"=w197) -> ("Preview"=→"Image":picture)  [unwired: 1 in]
        n70 = Enqueue Element(queue=w208, element=cluster{"State":string, "Data":variant} {"State"="Analyze Image", "Data"=variant}, error in (no error)=w189) -> (error out=w209:errorcluster)  [unwired: 1 in, 2 out]
        "Frame" <- w200
      }
      frame "Analyze Image" {
        # "simple brightness mean, SD\ncalc on image data."
        # "Run analysis on current image"
        n71 = call <vilib>:"Std Deviation and Variance.vi"("X"=w221) -> ("mean"=w219:dbl, "standard deviation"=w220:dbl)  [unwired: 1 in, 1 out]
        n72 = Format Into String(format string="%.02f +/- %.02f DN", w219, w220) -> (resulting string=→"Frame Brightness":string)  [unwired: 2 in, 1 out]
        n73 = Greater Or Equal?(x=w225, y=w224) -> (x >= y?=w226:bool)
        n74 = case shown="False" w226 {
          tunnel: w230 -> [w234 w235]
          tunnel: [w233 w235] -> w228
          tunnel: w227 -> [w232 _]
          frame False {
            # "get next image"
            n75 = Enqueue Element(queue=w232, element=cluster{"State":string, "Data":variant} {"State"="Get Image", "Data"=variant}, error in (no error)=w234) -> (error out=w233:errorcluster)  [unwired: 1 in, 2 out]
          }
          frame True {
            # "all done."
          }
        }
        n76 = Increment(x=w225) -> (x+1=w223:i32)
      }
      frame "Save" {
        # "save c1 to disk using SDK save dialog"
        n77 = call "Vision Research Phantom Series PhFile PhNewCineFromCamera.vi"("Camera Number in"=w247, "CineNr in"=1, "Error In (no error)"=w248) -> ("pCH"=w244:u32, "Error Out"=w245:errorcluster)  [unwired: 1 in, 14 out]
        n78 = call "Vision Research Phantom Series PhFile PhGetSaveCineName.vi"("CH in"=w244, "Error In (no error)"=w245) -> ("CH out"=w241:u32, "Success"=w240:bool, "Error Out"=w243:errorcluster)  [unwired: 15 out]
        n79 = case shown="True" w240 {
          tunnel: w243 -> [w249 w255]
          tunnel: [w249 w254] -> w242
          tunnel: w241 -> [_ w252]
          frame False {
            # "not success, don't save."
          }
          frame True {
            # "locks here\nuntil save complete"
            n80 = call "Vision Research Phantom Series PhFile PhWriteCineFile.vi"("CH in"=w252, "Error In (no error)"=w255) -> ("CH out"=w256:u32, "Error Out"=w250:errorcluster)  [unwired: 1 in, 15 out]
            n81 = Obtain Notifier(notification data type=FALSE) -> (notifier out=w251:refnum<notifier>)  [unwired: 3 in, 2 out]
            n82 = while {
              tunnel: w251 -> [w262]
              tunnel: [w259] -> _
              tunnel: w252 -> [w258]
              stop <- w260 stop-if-true
              n83 = Wait on Notification(notifier=w262, timeout in ms (-1)=500) -> (error out=w260:errorcluster)  [unwired: 2 in, 3 out]
              n84 = call "Vision Research Phantom Series PhFile PhGetWriteCineFileProgress.vi"("CH [in]"=w258, "Error In (no error)"=w260) -> ("pProgressPercent [out]"=→"Progress":u32, "Error Out"=w259:errorcluster)  [unwired: 16 out]
            }
            n85 = Release Notifier(notifier=w251, error in (no error)=w250) -> ()  [unwired: 1 in, 3 out]
            n86 = call "Vision Research Phantom Series PhFile PhDestroyCine.vi"("CH in"=w256, "Error In (no error)"=w250) -> ("Error Out"=w254:errorcluster)  [unwired: 17 out]
          }
        }
      }
      frame "Show Help" {
        # "opens up the LabVIEW SDK help pdf"
        n87 = VI Library() -> (path=w266:path)
        n88 = Strip Path(path=w266) -> (stripped path=w265:path)  [unwired: 1 out]
        n89 = Build Path(base path=w265, name or relative path="instr.lib\\Vision Research Phantom Series Labview Driver\\Phantom SDK Reference Manual.pdf") -> (appended path=w263:path)
        n90 = call-poly <vilib>:"Open URL in Default Browser.vi"("error in (no error)"=w273, "path"=w263) -> ("error out"=w272:errorcluster)  [unwired: 4 in, 1 out]
      }
      frame "Error" {
        # "Error happened. Display and clear."
        n91 = call <vilib>:"Simple Error Handler.vi"("error in (no error)"=w281) -> ("error out"=w280:errorcluster)  [unwired: 4 in, 4 out]
        n92 = call <vilib>:"Clear Errors.vi"("error in (no error)"=w280) -> ("error out"=w279:errorcluster)  [unwired: 6 in]
      }
      frame "Stop" {
        # "Stop this loop and all other loops"
        n93 = Generate User Event(user event=w294, event data cluster=cluster{"State":string, "Data":variant} {"State"="Stop", "Data"=variant} ("event data"), error in=w290) -> (error out=w292:errorcluster)  [unwired: 1 in, 1 out]
        n94 = Release Queue(queue=w286, error in (no error)=w292) -> (error out=w287:errorcluster)  [unwired: 1 in, 2 out]
        n95 = call <vilib>:"Clear Errors.vi"("error in (no error)"=w287) -> ("error out"=w291:errorcluster)  [unwired: 6 in]
        n96 = call "Vision Research Phantom Series Close.vi"("Error In (no error)"=w291) -> ("Error Out"=w289:errorcluster)  [unwired: 18 out]
      }
    }
  }
  n97 = while "Producer Loop" {
    tunnel: w12 -> [w300]
    shift-right: [w298] -> _
    shift-left: w10 -> [w299]
    tunnel: w17 -> [w297]
    tunnel: [w296] -> w16
    stop <- w301 stop-if-true
    n98 = event shown="[0] Panel Close?" {
      selector: w297 -> [_ _ _ _ _ _ _ _ _]
      dyn-events: [_ _ _ _ _ _ _ _ _] -> w296
      timeout: _ -> [_ _ _ _ _ _ _ _ _]
      tunnel: [w306 w310 _ _ _ _ _ _ _] -> w301
      tunnel: w300 -> [w303 _ w318 w322 w326 w331 w334 w339 w342]
      tunnel: w299 -> [w305 w307 w320 w324 w328 w329 w336 w337 w344]
      tunnel: [w304 w308 w319 w323 w327 w332 w335 w340 w343] -> w298
      event Panel Close? {
        w306 = TRUE ("Discard?")
        n99 = event-data() -> ()  [unwired: 1 in, 1 out]
        n100 = Enqueue Element At Opposite End(queue=w303, element=cluster{"State":string, "Data":variant} {"State"="Stop", "Data"=variant}, error in (no error)=w305) -> (error out=w304:errorcluster)  [unwired: 1 in, 2 out]
        n101 = event-data("Discard?"=w306) -> ()  [unwired: 1 in, 1 out]
      }
      event User Event {
        n102 = event-data() -> ("State"=w311:string, "Data"=w309:variant)  [unwired: 1 in]
        n103 = case shown="Default" w311 {
          tunnel: [_ TRUE] -> w310
          tunnel: w309 -> [_ _]
          tunnel: [w312 w313] -> w308
          tunnel: w307 -> [w312 w313]
          frame Default {
          }
          frame "Stop" {
          }
        }
      }
      event "Camera Number": Value Change {
        n104 = event-data() -> ()  [unwired: 1 in, 1 out]
        n105 = Bundle By Name(cluster=cluster{"State":string, "Data":variant} {"State"="Get Cam Info", "Data"=variant} ("element"), "Data"="Camera Number") -> (w316:cluster{"State":string, "Data":variant})
        n106 = Enqueue Element(queue=w318, element=w316, error in (no error)=w320) -> (error out=w319:errorcluster)  [unwired: 1 in, 2 out]
      }
      event "Res", "Rate", "Exp": Value Change {
        n107 = event-data() -> ()  [unwired: 1 in, 1 out]
        n108 = Enqueue Element(queue=w322, element=cluster{"State":string, "Data":variant} {"State"="Update Settings", "Data"=variant}, error in (no error)=w324) -> (error out=w323:errorcluster)  [unwired: 1 in, 2 out]
      }
      event "Help": Value Change {
        n109 = event-data() -> ()  [unwired: 1 in, 1 out]
        n110 = Enqueue Element(queue=w326, element=cluster{"State":string, "Data":variant} {"State"="Show Help", "Data"=variant}, error in (no error)=w328) -> (error out=w327:errorcluster)  [unwired: 1 in, 2 out]
      }
      event "Record": Value Change {
        n111 = event-data() -> ()  [unwired: 1 in, 1 out]
        n112 = Enqueue Element(queue=w331, element=cluster{"State":string, "Data":variant} {"State"="Record", "Data"=variant}, error in (no error)=w329) -> (error out=w332:errorcluster)  [unwired: 1 in, 2 out]
      }
      event "Trigger": Value Change {
        n113 = event-data() -> ()  [unwired: 1 in, 1 out]
        n114 = Enqueue Element(queue=w334, element=cluster{"State":string, "Data":variant} {"State"="Trigger", "Data"=variant}, error in (no error)=w336) -> (error out=w335:errorcluster)  [unwired: 1 in, 2 out]
      }
      event "Playback": Value Change {
        n115 = event-data() -> ()  [unwired: 1 in, 1 out]
        n116 = Enqueue Element(queue=w339, element=cluster{"State":string, "Data":variant} {"State"="Start Playback", "Data"=variant}, error in (no error)=w337) -> (error out=w340:errorcluster)  [unwired: 1 in, 2 out]
      }
      event "Save": Value Change {
        n117 = event-data() -> ()  [unwired: 1 in, 1 out]
        n118 = Enqueue Element(queue=w342, element=cluster{"State":string, "Data":variant} {"State"="Save", "Data"=variant}, error in (no error)=w344) -> (error out=w343:errorcluster)  [unwired: 1 in, 2 out]
      }
    }
  }
  n119 = Unregister For Events(event registration refnum=w16) -> (error out=w15:errorcluster)  [unwired: 1 in]
  n120 = Destroy User Event(user event=w13, error in=w15) -> (error out=w14:errorcluster)
  n121 = call <vilib>:"Clear Errors.vi"("error in (no error)"=w14) -> ()  [unwired: 6 in, 1 out]
